vi "AOwrite_set_trig_v4.vi"(0 "AO Channels":refnum<k21>[](array[refnum])=["AO0_0", "AO0_1", "AO0_2", "AO0_3"], 1 "DO Channel":refnum<k21>="DO0", 2 "Pause.DigLvl.Src":tag="/Dev2/PFI1", 3 "AI Channels":refnum<k21>[](array[refnum])=["AO0_0", "AO0_1", "AO0_2", "AO0_3"], 4 "Pulse terminal":tag="/Dev1/PFI3", 5 "AO Data array":dbl[][](array[numeric])=[[0.0, 0.0, 0.0, 1.0]], 7 "AI Sample Rate":dbl, 9 "DO Data array":bool[][](array[boolean])=[[TRUE, TRUE, TRUE, TRUE, TRUE, TRUE, TRUE, TRUE, TRUE, TRUE, TRUE, TRUE, TRUE, TRUE, TRUE, TRUE]], 11 "error in":errorcluster, 12 "Source terminal":tag="/Dev1/PFI0", 13 "active edge":i32(ring)=10280 items=["Rising"=10280, "Falling"=10171], 14 "Total Time":dbl) -> (6 "AI Task Out":refnum<k21>, 10 "Tasks Out":refnum<k21>[](array[refnum]), 15 "error out":errorcluster={"status"=TRUE, "code"=-200077, "source"="DAQmx Write (Analog 2D DBL NChan NSamp).vi:1<append>\n<B>Property: </B>SampQuant.SampPerChan\n<B>You Have Requested: </B>1\n<B>Valid Values Begin with: </B>2\n<B>Valid Values End with: </B>18446744065119617024\n\n<B>Task Name: </B>_unnamedTask<C>"})   [LabVIEW 2013]
uses:
  <vilib>/DAQmx/write.llb/DAQmx Write.vi
  <vilib>/DAQmx/write.llb/DAQmx Write (Digital 1D U32 1Chan NSamp).vi
  <vilib>/DAQmx/write.llb/DAQmx Write (Digital 1D U16 1Chan NSamp).vi
  <vilib>/DAQmx/write.llb/DAQmx Write (Digital 1D U8 1Chan NSamp).vi
  <vilib>/DAQmx/write.llb/DAQmx Write (Analog 2D DBL NChan NSamp).vi
  <vilib>/DAQmx/configure/timing.llb/DAQmx Timing (Sample Clock).vi
  <vilib>/DAQmx/configure/trigger.llb/DAQmx Start Trigger (Digital Edge).vi
  <vilib>/DAQmx/miscellaneous.llb/DAQmx Fill In Error Info.vi
  <resource>/objmgr/daqmx.rc
panel:
  out "error out 2":errorcluster={"status"=TRUE, "code"=-200077, "source"="DAQmx Write (Analog 2D DBL NChan NSamp).vi:1<append>\n<B>Property: </B>SampQuant.SampPerChan\n<B>You Have Requested: </B>1\n<B>Valid Values Begin with: </B>2\n<B>Valid Values End with: </B>18446744065119617024\n\n<B>Task Name: </B>_unnamedTask<C>"}
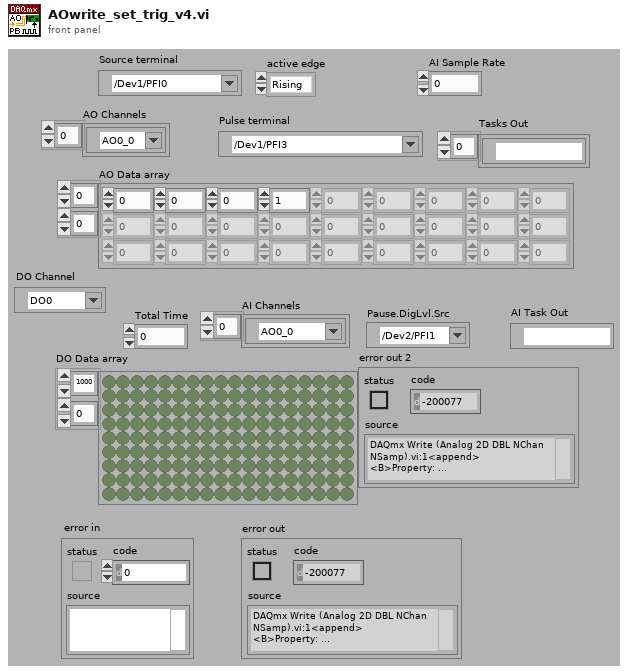
[diagram p1: front panel]
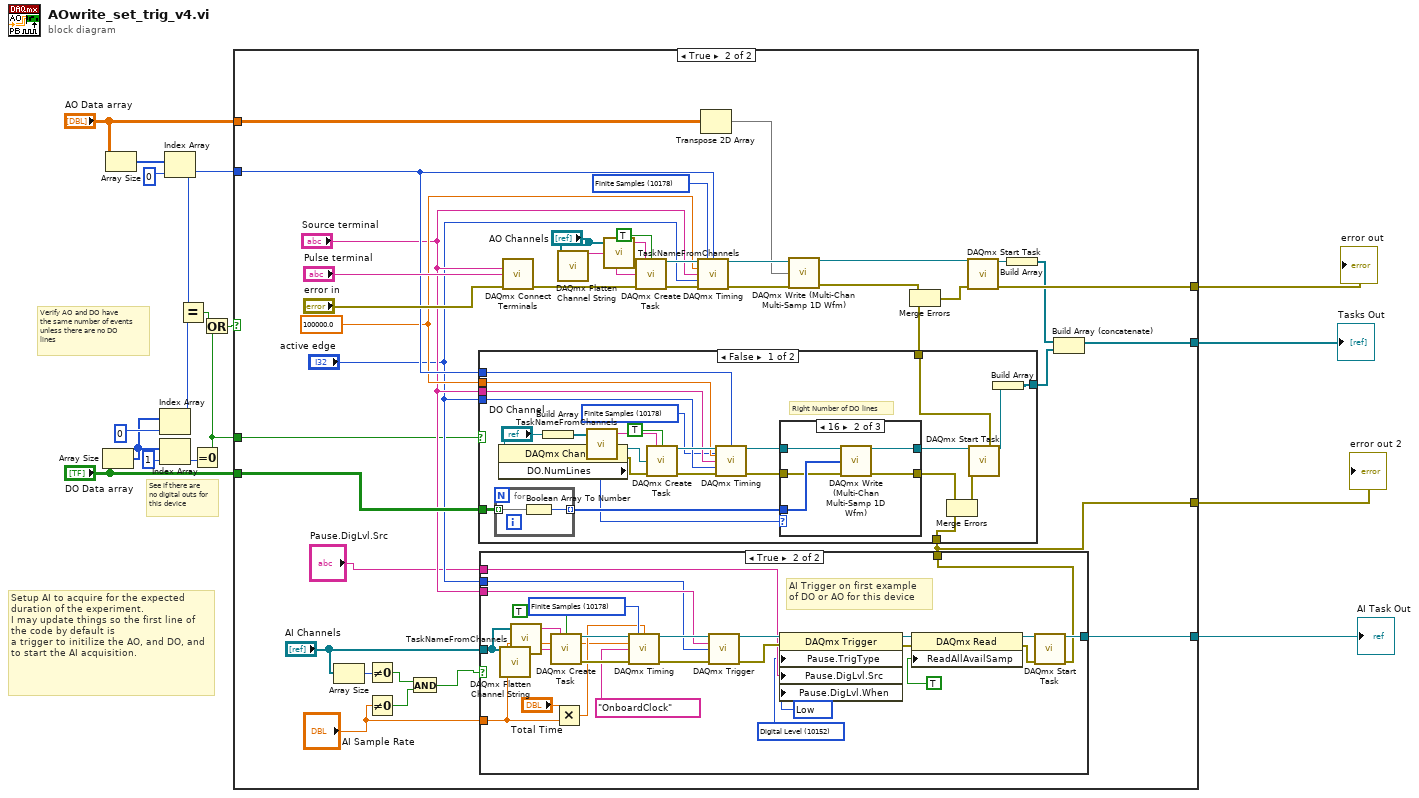
[diagram p0: block diagram]
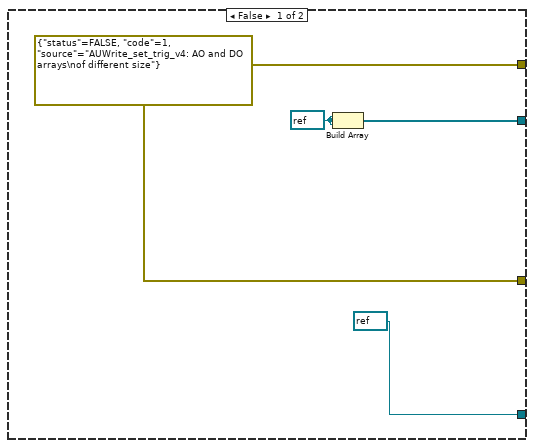
[diagram p2: hidden frame]
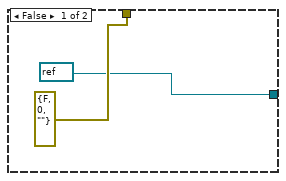
[diagram p3: hidden frame]
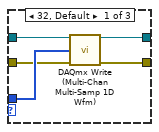
[diagram p4: hidden frame]
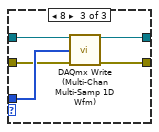
[diagram p5: hidden frame]
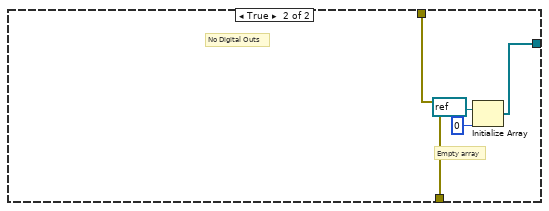
[diagram p6: hidden frame]
diagram:
  # "Setup AI to acquire for the expected duration of the experiment.\nI may update things so the first line of the code by default is\na trigger to initilize the AO, and DO, and to start the AI acquisition."
  # "Verify AO and DO have \nthe same number of events\nunless there are no DO\nlines"
  # "See if there are\nno digital outs for\nthis device"
  n1 = Array Size(array="DO Data array") -> (size(s)=w5:i32[])
  n2 = Array Size(array="AO Data array") -> (size(s)=w16:i32[])
  n3 = Index Array(array=w5, index=0) -> (element=w12:i32)
  n4 = Index Array(array=w5, index=1) -> (element=w3:i32)
  n5 = Index Array(array=w16, index=0) -> (element=w11:i32)
  n6 = Equal?(x=w11, y=w12) -> (x = y?=w7:bool)
  n7 = Equal To 0?(x=w3) -> (x = 0?=w2:bool)
  n8 = Or(x=w7, y=w2) -> (x .or. y?=w6:bool)
  n9 = case shown="True" w6 {
    tunnel: "AO Data array" -> [_ w57]
    tunnel: w11 -> [_ w44]
    tunnel: "DO Data array" -> [_ w47]
    tunnel: [w20 w50] -> w10
    tunnel: [refnum<k21> refnum ("AO task out") w42] -> w9
    tunnel: [w20 w31] -> w8
    tunnel: w2 -> [_ w38]
    tunnel: [w19 w36] -> w1
    frame False {
      w20 = errorcluster {"status"=FALSE, "code"=1, "source"="AUWrite_set_trig_v4: AO and DO arrays\nof different size"} ("error out")
      w18 = refnum<k21> refnum ("AO task out")
      n10 = Build Array(w18, w18) -> (w19:refnum<k21>[])
    }
    frame True {
      w43 = 100000.0 ("rate")
      w39 = 10178 items=["Finite Samples"=10178, "Continuous Samples"=10123, "Hardware Timed Single Point"=12522] ("sample mode")
      n11 = Array Size(array="AI Channels") -> (size(s)=w32:i32)
      n12 = Not Equal To 0?(x=w32) -> (x != 0?=w29:bool)
      n13 = Not Equal To 0?(x="AI Sample Rate") -> (x != 0?=w27:bool)
      n14 = And(x=w29, y=w27) -> (x .and. y?=w28:bool)
      n15 = case shown="True" w28 {
        tunnel: [refnum<k21> refnum ("task out") w84] -> w42
        tunnel: "Source terminal" -> [_ w79]
        tunnel: "active edge" -> [_ w78]
        tunnel: "AI Channels" -> [_ w63]
        tunnel: [errorcluster {"status"=FALSE, "code"=0, "source"=""} ("error out") w77] -> w31
        tunnel: "Pause.DigLvl.Src" -> [_ w68]
        tunnel: "AI Sample Rate" -> [_ w65]
        frame False {
        }
        frame True {
          w66 = 10214 items=["High"=10192, "Low"=10214] ("Pause.DigLvl.When")
          w67 = 10152 items=["Analog Level"=10101, "Analog Window"=10103, "Digital Level"=10152, "Digital Pattern"=10398, "None"=10230] ("Pause.TrigType")
          w83 = 10178 items=["Finite Samples"=10178, "Continuous Samples"=10123, "Hardware Timed Single Point"=12522] ("sample mode")
          # "AI Trigger on first example\nof DO or AO for this device"
          n16 = call <vilib>:"DAQmx Flatten Channel String.vi"("names in"=w63) -> ("names out"=w88:string)  [unwired: 1 in, 13 out]
          n17 = call "TaskNameFromChannels.vi"("I/O Channels"=w63) -> ("Task Name"=w64:string)  [unwired: 4 in]
          n18 = call <vilib>:"DAQmx Create Task.vi"("new task name"=w64, "auto cleanup"=TRUE, "global virtual channels"=w88) -> ("task out"=w86:refnum<k21>, "error out"=w87:errorcluster)  [unwired: 2 in, 9 out]
          n19 = Multiply(x="Total Time", y=w65) -> (x*y=w69:dbl)
          n20 = call-poly <vilib>:"DAQmx Timing.vi"("task/channels in"=w86, "sample mode"=w83, "samples per channel"=w69, "rate"=w65, "source"=tag "OnboardClock", "error in"=w87) -> ("task out"=w80:refnum<k21>, "error out"=w81:errorcluster)  [unwired: 1 in, 7 out]
          n21 = call-poly <vilib>:"DAQmx Trigger.vi"("task/channels in"=w80, "source"=w79, "edge"=w78, "error in"=w81) -> ("task out"=w76:refnum<k21>, "error out"=w75:errorcluster)  [unwired: 1 in, 9 out]
          n22 = property class="DAQmx Trigger"(reference=w76, error in=w75, "Pause.TrigType"=w67, "Pause.DigLvl.Src"=w68, "Pause.DigLvl.When"=w66) -> (reference out=w74:refnum<k21>, error out=w73:errorcluster)
          n23 = property class="DAQmx Read"(reference=w74, error in=w73, "ReadAllAvailSamp"=TRUE) -> (reference out=w72:refnum<k21>, error out=w71:errorcluster)
          n24 = call <vilib>:"DAQmx Start Task.vi"("task/channels in"=w72, "error in"=w71) -> ("task out"=w84:refnum<k21>, "error out"=w77:errorcluster)  [unwired: 12 out]
        }
      }
      n25 = case shown="False" w38 {
        tunnel: [w97 w133] -> w34
        tunnel: [w113 w134] -> w48
        tunnel: w47 -> [w112 _]
        tunnel: w44 -> [w106 _]
        tunnel: w43 -> [w105 _]
        tunnel: w31 -> [w102 w134]
        tunnel: "Source terminal" -> [w101 _]
        tunnel: "active edge" -> [w100 _]
        frame False {
          w99 = 10178 items=["Finite Samples"=10178, "Continuous Samples"=10123, "Hardware Timed Single Point"=12522] ("sample mode")
          # "Right Number of DO lines"
          n26 = for {
            tunnel: w112 -> [w130] mode=indexing
            tunnel: [w129] -> w111 mode=indexing
            n27 = Boolean Array To Number(Boolean array=w130) -> (number=w129:u32)
          }
          n28 = property class="DAQmx Channel"(reference="DO Channel") -> (reference out=w95:refnum<k21>, error out=w94:errorcluster, "DO.NumLines"=w93:u32)  [unwired: 1 in]
          n29 = Build Array("DO Channel") -> (w90:refnum<k21>[])
          n30 = call "TaskNameFromChannels.vi"("I/O Channels"=w90) -> ("Task Name"=w92:string)  [unwired: 4 in]
          n31 = call <vilib>:"DAQmx Create Task.vi"("new task name"=w92, "auto cleanup"=TRUE, "global virtual channels"=w95, "error in"=w94) -> ("task out"=w107:refnum<k21>, "error out"=w108:errorcluster)  [unwired: 1 in, 9 out]
          n32 = call-poly <vilib>:"DAQmx Timing.vi"("task/channels in"=w107, "sample mode"=w99, "samples per channel"=w106, "rate"=w105, "source"=w101, "active edge"=w100, "error in"=w108) -> ("task out"=w96:refnum<k21>, "error out"=w110:errorcluster)  [unwired: 7 out]
          n33 = case shown="16" w93 {
            tunnel: w111 -> [w118 w123 w128]
            tunnel: w110 -> [w117 w122 w127]
            tunnel: [w116 w121 w126] -> w109
            tunnel: [w115 w120 w125] -> w104
            tunnel: w96 -> [w114 w119 w124]
            frame 32, Default {
              n34 = call-poly "DAQmx Write (Multi-Chan Multi-Samp 1D Wfm).vi"("task/channels in"=w114, "data"=w118, "error in"=w117) -> ("task out"=w116:refnum<k21>, "error out"=w115:errorcluster)  [unwired: 1 in, 10 out]
            }
            frame 16 {
              n35 = call-poly "DAQmx Write (Multi-Chan Multi-Samp 1D Wfm).vi"("task/channels in"=w119, "data"=w123, "error in"=w122) -> ("task out"=w121:refnum<k21>, "error out"=w120:errorcluster)  [unwired: 1 in, 10 out]
            }
            frame 8 {
              n36 = call-poly "DAQmx Write (Multi-Chan Multi-Samp 1D Wfm).vi"("task/channels in"=w124, "data"=w128, "error in"=w127) -> ("task out"=w126:refnum<k21>, "error out"=w125:errorcluster)  [unwired: 1 in, 10 out]
            }
          }
          n37 = Merge Errors(w104, w102) -> (w103:errorcluster)
          n38 = call <vilib>:"DAQmx Start Task.vi"("task/channels in"=w109, "error in"=w103) -> ("task out"=w98:refnum<k21>, "error out"=w113:errorcluster)  [unwired: 12 out]
          n39 = Build Array(w98) -> (w97:refnum<k21>[])
        }
        frame True {
          # "Empty array"
          # "No Digital Outs"
          n40 = Initialize Array(refnum<k21> refnum ("task out"), 0 ("dimension size")) -> (w133:refnum<k21>[])
        }
      }
      n41 = call <vilib>:"DAQmx Connect Terminals.vi"("source terminal"="Source terminal", "destination terminal"="Pulse terminal", "error in"="error in") -> ("error out"=w52:errorcluster)  [unwired: 1 in, 11 out]
      n42 = call <vilib>:"DAQmx Flatten Channel String.vi"("names in"="AO Channels") -> ("names out"=w25:string)  [unwired: 1 in, 13 out]
      n43 = call "TaskNameFromChannels.vi"("I/O Channels"="AO Channels") -> ("Task Name"=w23:string)  [unwired: 4 in]
      n44 = call <vilib>:"DAQmx Create Task.vi"("new task name"=w23, "auto cleanup"=TRUE, "global virtual channels"=w25, "error in"=w52) -> ("task out"=w55:refnum<k21>, "error out"=w56:errorcluster)  [unwired: 1 in, 9 out]
      n45 = call-poly <vilib>:"DAQmx Timing.vi"("task/channels in"=w55, "sample mode"=w39, "samples per channel"=w44, "rate"=w43, "source"="Source terminal", "active edge"="active edge", "error in"=w56) -> ("task out"=w59:refnum<k21>, "error out"=w58:errorcluster)  [unwired: 7 out]
      n46 = Transpose 2D Array(2D array=w57) -> (transposed array=w54:dbl[][])
      n47 = call-poly "DAQmx Write (Multi-Chan Multi-Samp 1D Wfm).vi"("task/channels in"=w59, "data"=w54, "error in"=w58) -> ("task out"=w45:refnum<k21>, "error out"=w46:errorcluster)  [unwired: 1 in, 10 out]
      n48 = Merge Errors(w46, w48) -> (w49:errorcluster)
      n49 = call <vilib>:"DAQmx Start Task.vi"("task/channels in"=w45, "error in"=w49) -> ("task out"=w37:refnum<k21>, "error out"=w50:errorcluster)  [unwired: 12 out]
      n50 = Build Array(w37) -> (w35:refnum<k21>[])
      n51 = Build Array (concatenate)(w35, w34) -> (w36:refnum<k21>[])
    }
  }
  "Tasks Out" <- w1
  "error out" <- w10
  "AI Task Out" <- w9
  "error out 2" <- w8
